vi "ApproveAllCoords (SubVI).vi"(8 "error in (no error)":errorcluster, 10 "Go to Coordinates":T1, 11 "Controller .NET Refnum in":refnum<k24>) -> (0 "error out":errorcluster, 2 "Approved Coordinates":T1, 3 "Controller .NET Refnum out":refnum<k24>)   [LabVIEW 2016]
uses:
  C:/Users/Aerotech/Documents/BNLStaveAssembly/Bin/Aerotech.A3200.dll
  Bin/Aerotech.A3200.dll
panel:
  in  "Zlow":dbl=-50.0 format="%#_13g"
  in  "Zhigh":dbl=50.0 format="%#_13g"
  in  "Ylow":dbl=-150.0 format="%#_13g"
  in  "Yhigh":dbl=30.0 format="%#_13g"
  in  "Xhigh":dbl=750.0 format="%#_13g"
  in  "Xlow":dbl=-750.0 format="%#_13g"
  # "Supply motion boundaries"
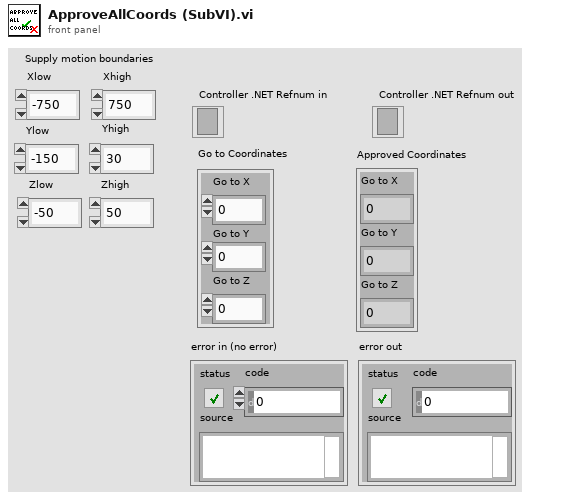
[diagram p1: front panel]
types:
  T1 = cluster{"Go to X":dbl, "Go to Y":dbl, "Go to Z":dbl}
  T2 = cluster{"X Position Feedback":dbl, "Y Position Feedback":dbl, "Z Position Feedback":dbl}
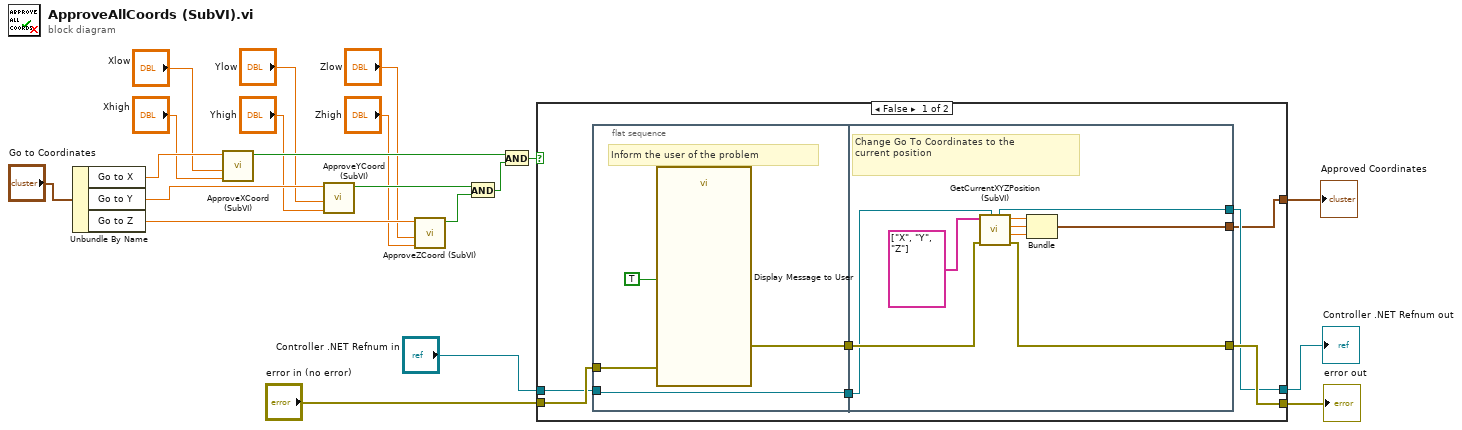
[diagram p0: block diagram]
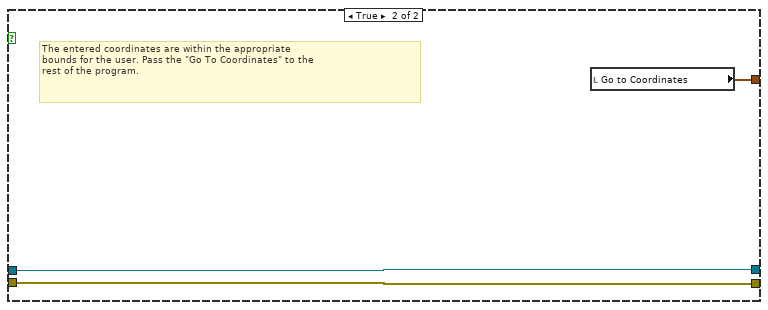
[diagram p2: hidden frame]
diagram:
  n1 = Unbundle By Name("Go to Coordinates") -> ("Go to X"=w9:dbl, "Go to Y"=w6:dbl, "Go to Z"=w10:dbl)
  n2 = call "ApproveXCoord (SubVI).vi"("Xhigh"="Xhigh", "Xlow"="Xlow", "Go to X"=w9) -> ("Pass X?"=w15:bool)  [unwired: 8 in]
  n3 = call "ApproveYCoord (SubVI).vi"("Yhigh"="Yhigh", "Ylow"="Ylow", "Go to Y"=w6) -> ("Pass Y?"=w13:bool)  [unwired: 8 in]
  n4 = call "ApproveZCoord (SubVI).vi"("Zhigh"="Zhigh", "Zlow"="Zlow", "Go to Z"=w10) -> ("Pass Z?"=w12:bool)  [unwired: 8 in]
  n5 = And(x=w13, y=w12) -> (x .and. y?=w14:bool)
  n6 = And(x=w15, y=w14) -> (x .and. y?=w16:bool)
  n7 = case shown="False" w16 {
    tunnel: "error in (no error)" -> [w27 w41]
    tunnel: [w25 w41] -> w17
    tunnel: "Controller .NET Refnum in" -> [w23 w43]
    tunnel: [w22 w43] -> w19
    tunnel: [w21 w42] -> w20
    frame False {
      n8 = flat-sequence {
        tunnel: w27 -> [w30]
        tunnel: [w29] -> w26
        tunnel: [w28] -> w24
        tunnel: w23 -> [w28]
        tunnel: [w35] -> w25
        tunnel: w26 -> [w36]
        tunnel: w24 -> [w34]
        tunnel: [w33] -> w22
        tunnel: [w32] -> w21
        frame #0 {
          # "Inform the user of the problem"
          n9 = call "Display Message to User"("error in (no error)"=w30, "Enable"=TRUE) -> ("error out"=w29:errorcluster)  [unwired: 8 in, 1 out]
        }
        frame #1 {
          # "Change Go To Coordinates to the\ncurrent position"
          n10 = call "GetCurrentXYZPosition (SubVI).vi"(".NET Refnum in - Device"=w34, "error in (no error)"=w36, "Axes Names"=string[] ["X", "Y", "Z"]) -> ("error out"=w35:errorcluster, "Z Position Feedback"=w37:dbl, "Y Position Feedback"=w38:dbl, "X Position Feedback"=w39:dbl, ".NET Refnum out  - Device"=w33:refnum<k24>)  [unwired: 3 in]
          n11 = Bundle("X Position Feedback"=w39, "Y Position Feedback"=w38, "Z Position Feedback"=w37) -> (w32:T2)  [unwired: 1 in]
        }
      }
    }
    frame True {
      # "The entered coordinates are within the appropriate\nbounds for the user. Pass the \"Go To Coordinates\" to the \nrest of the program."
      n12 = local read "Go to Coordinates"() -> (w42:T1)
    }
  }
  "Approved Coordinates" <- w20
  "Controller .NET Refnum out" <- w19
  "error out" <- w17
